vi "Read Current Count.vi"(8 "error in (no error)":errorcluster, 11 "Complex in":refnum<class "Complex.lvclass">) -> (0 "error out":errorcluster, 2 "Current Count":cdb, 3 "Complex out":refnum<class "Complex.lvclass">)   [LabVIEW 2018, in "Complex.lvclass"]
uses:
  Complex.lvclass
  Complex.lvclass/Complex.ctl
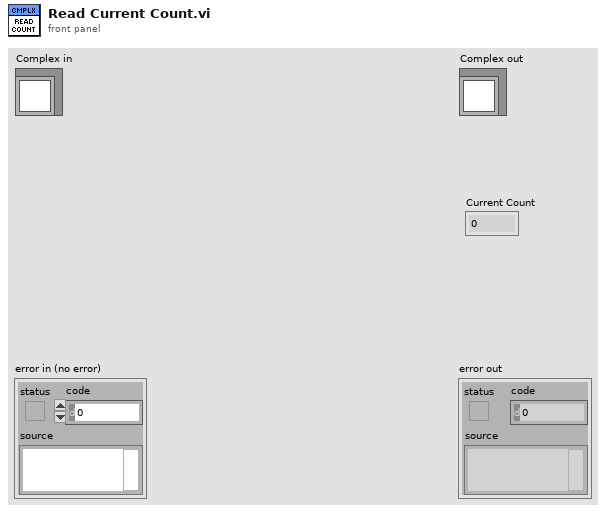
[diagram p1: front panel]
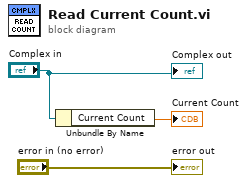
[diagram p0: block diagram]
diagram:
  n1 = Unbundle By Name("Complex in") -> ("Current Count"=→"Current Count":cdb)
  "error out" <- "error in (no error)"
  "Complex out" <- "Complex in"
